vi "ColorSlider.vi"(8 "error in (no error)":errorcluster, 9 "slider_background 2":refnum<vi>, 10 "slider_background":refnum<vi>, 11 "PredictiveMaintenance in":refnum<class "PredictiveMaintenance.lvclass">) -> (0 "error out":errorcluster, 3 "PredictiveMaintenance OUT":refnum<class "PredictiveMaintenance.lvclass">)   [LabVIEW 2019, in "PredictiveMaintenance.lvlib" / "PredictiveMaintenance.lvclass"]
uses:
  PredictiveMaintenance.lvclass
  PredictiveMaintenance.lvclass/PredictiveMaintenance.ctl
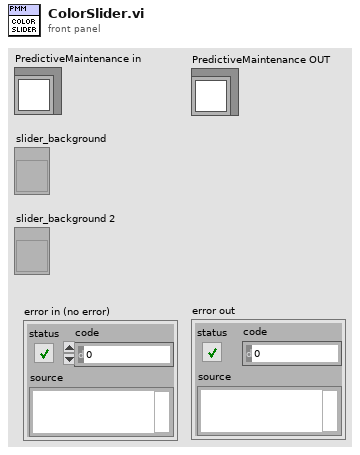
[diagram p1: front panel]
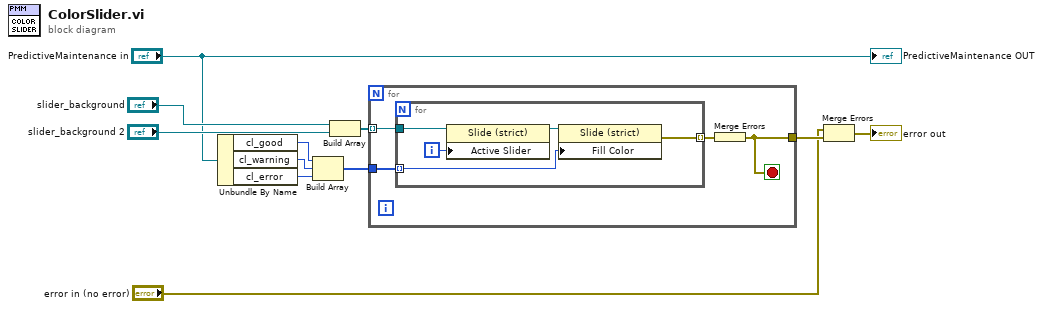
[diagram p0: block diagram]
diagram:
  n1 = Unbundle By Name("PredictiveMaintenance in") -> ("cl_good"=w10:u32, "cl_warning"=w11:u32, "cl_error"=w7:u32)
  n2 = Build Array(w10, w11, w7) -> (w6:u32[])
  n3 = Build Array("slider_background", "slider_background 2") -> (w8:refnum<vi>[])
  n4 = for {
    tunnel: w8 -> [w15] mode=indexing
    tunnel: w6 -> [w14]
    tunnel: [w12] -> w3
    stop <- w12 stop-if-true
    n5 = for {
      tunnel: w15 -> [w20]
      tunnel: w14 -> [w17] mode=indexing
      tunnel: [w16] -> w13 mode=indexing
      i -> [w19]
      n6 = property class="Slide (strict)"(reference=w20, "Active Slider"=w19) -> (reference out=w18:refnum<vi>)  [unwired: 1 in, 1 out]
      n7 = property class="Slide (strict)"(reference=w18, "Fill Color"=w17) -> (error out=w16:errorcluster)  [unwired: 1 in, 1 out]
    }
    n8 = Merge Errors(w13) -> (w12:errorcluster)
  }
  n9 = Merge Errors("error in (no error)", w3) -> (→"error out":errorcluster)
  "PredictiveMaintenance OUT" <- "PredictiveMaintenance in"
